vi "WriteCommandToPort.vi"(8 "Error In":errorcluster, 10 "Command":string="R01", 11 "Omega CSi32 In":refnum<visa-resource-name>) -> (0 "Error Out":errorcluster, 3 "Omega CSi32 Out":refnum<visa-resource-name>)   [LabVIEW 2012, in "Omega-CSi32.lvlib"]
uses:
  Omega-CSi32.lvlib
  <vilib>/Instr/_visa.llb/VISA Flush IO Buffer Mask.ctl
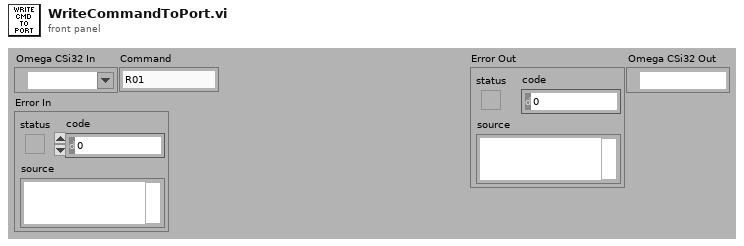
[diagram p1: front panel]
types:
  T1 = typedef "VISA Flush IO Buffer Mask.ctl" = u16
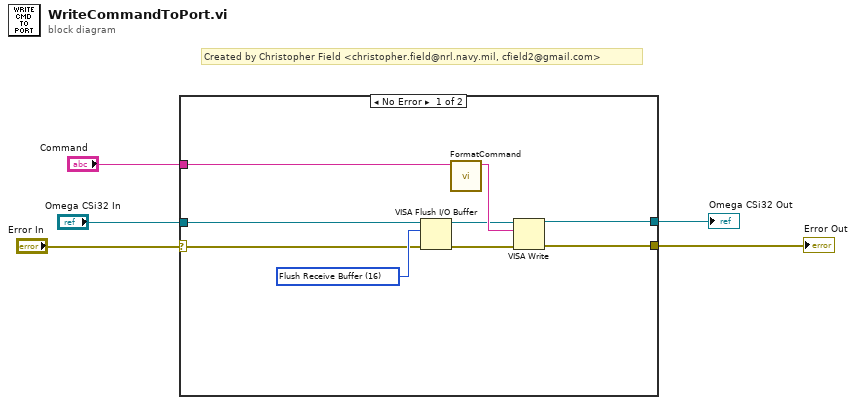
[diagram p0: block diagram]
diagram:
  # "Created by Christopher Field <christopher.field@nrl.navy.mil, cfield2@gmail.com>"
  n1 = case shown="No Error" "Error In" {
    selector: "Error In" -> [w6 w15]
    tunnel: "Command" -> [w14 _]
    tunnel: "Omega CSi32 In" -> [w9 w16]
    tunnel: [w8 w15] -> w3
    tunnel: [w7 w16] -> w2
    frame No Error {
      w10 = T1 16 items=["Flush Receive Buffer"=16, "Write Transmit Buffer to Device"=32, "Flush Receive Buffer (No I/O)"=64, "Flush Transmit Buffer"=128] ("Mask")
      n2 = VISA Flush I/O Buffer(VISA resource name=w9, mask (16)=w10, error in (no error)=w6) -> (VISA resource name out=w12:refnum<visa-resource-name>, error out=w11:errorcluster)
      n3 = call "FormatCommand.vi"("Command"=w14) -> ("Formatted Command"=w13:string)  [unwired: 10 in]
      n4 = VISA Write(VISA resource name=w12, write buffer=w13, error in (no error)=w11) -> (VISA resource name out=w7:refnum<visa-resource-name>, error out=w8:errorcluster)  [unwired: 1 out]
    }
    frame Error {
    }
  }
  "Error Out" <- w3
  "Omega CSi32 Out" <- w2
